vi "Serial Read Buffer Labview Community Ed.vi"() -> ()   [LabVIEW 2022 SP3]
uses:
  <vilib>/Instr/_visa.llb/VISA Configure Serial Port (Instr).vi
panel:
  out "read buffer":string
  in  "stop":bool
  in  "VISA resource name":refnum<visa-resource-name>
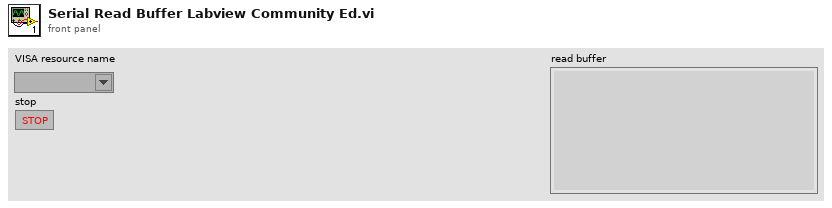
[diagram p1: front panel]
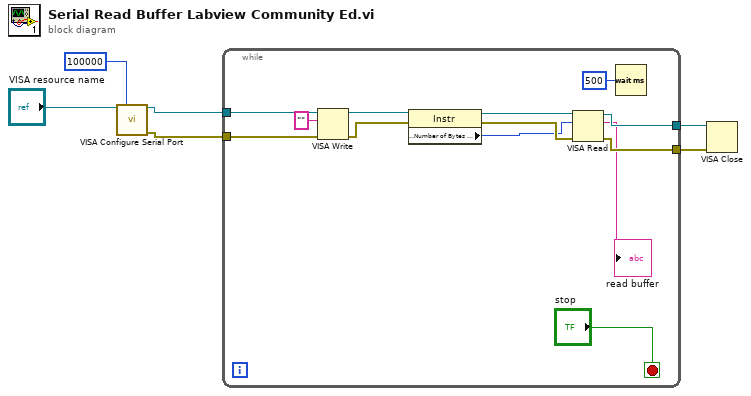
[diagram p0: block diagram]
diagram:
  n1 = call-poly "VISA Configure Serial Port"("VISA resource name"="VISA resource name", "timeout (10sec)"=u32 100000) -> ("VISA resource name out"=w4:refnum<visa-resource-name>, "error out"=w3:errorcluster)  [unwired: 12 in]
  n2 = while {
    tunnel: w4 -> [w19]
    tunnel: w3 -> [w18]
    tunnel: [w15] -> w2
    tunnel: [w13] -> w1
    stop <- "stop" stop-if-true
    n3 = VISA Write(VISA resource name=w19, write buffer="", error in (no error)=w18) -> (VISA resource name out=w17:refnum<visa-resource-name>, error out=w9:errorcluster)  [unwired: 1 out]
    n4 = property class="Instr"(reference=w17, error in=w9) -> (reference out=w16:refnum<visa-resource-name>, error out=w14:errorcluster, "Serial Settings:Number of Bytes at Serial Port"=w7:u32)
    n5 = VISA Read(VISA resource name=w16, byte count=w7, error in (no error)=w14) -> (VISA resource name out=w15:refnum<visa-resource-name>, read buffer=→"read buffer":string, error out=w13:errorcluster)  [unwired: 1 out]
    n6 = Wait (ms)(milliseconds to wait=u32 500) -> ()  [unwired: 1 out]
  }
  n7 = VISA Close(VISA resource name=w2, error in (no error)=w1) -> ()  [unwired: 1 out]
